vi "Configure Session.vi"(8 "error in":errorcluster, 11 "Plugin in":refnum<class "Sequencer with Output Values.lvclass">) -> (0 "error out":errorcluster, 3 "Plugin out":refnum<class "Sequencer with Output Values.lvclass">)   [LabVIEW 2024, in "Sequencer with Output Values.lvlib" / "Sequencer with Output Values.lvclass"]
uses:
  Sequencer with Output Values.lvclass
  C:/Program Files/National Instruments/LabVIEW 2024/vi.lib/FlexLogger/SDK/PluginSDK.lvlibp/PEFClasses/SDK/Processing Element/Processing Element.lvclass
  C:/Program Files/National Instruments/LabVIEW 2024/vi.lib/FlexLogger/SDK/PluginSDK.lvlibp/PEFClasses/SDK/Plugin/Plugin.lvclass
  Sequencer with Output Values.lvclass/Sequencer with Output Values.ctl
  <vilib>/FlexLogger/SDK/PluginSDK.lvlibp/PEFClasses/SDK/Producer Channel/Producer Channel.lvclass
  C:/Program Files/National Instruments/LabVIEW 2024/vi.lib/FlexLogger/SDK/PluginSDK.lvlibp/PEFClasses/SDK/Channel/Channel.lvclass
  <vilib>/FlexLogger/SDK/PluginSDK.lvlibp/PEFClasses/SDK/Processing Element/Read Alias.vi
  Global Strings.vi
  <vilib>/FlexLogger/SDK/PluginSDK.lvlibp/PEFClasses/SDK/Plugin/ParameterAccess/Read String.vi
  <vilib>/FlexLogger/SDK/PluginSDK.lvlibp/PEFClasses/SDK/Plugin/Plugin.lvclass
  C:/dev/niflexlogger-plugins/plugins/Sequencer with Output Values/source/Sequencer with Output Values/Sequencer with Output Values.lvclass
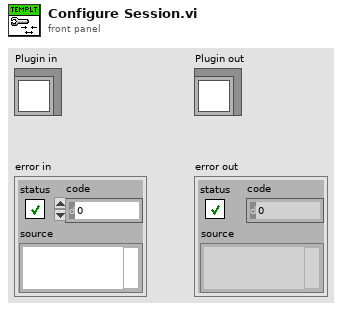
[diagram p1: front panel]
types:
  T1 = typedef "Sequencer with Output Values.lvlib/Sequencer with Output Values.lvclass/Params.ctl" = cluster{"Step Values":T2[], "Only Execute When Test Running":bool, "Reset Sequence When Test Starts":bool, "Current Sequence ID":u32, "Total Iterations":u32, "Current Step Start Timestamp":dbl, "Number of Sequence Steps":i32, "Num of Analog Channels":i32, "Num of Digital Channels":i32, "Delay Before Starting Sequence":dbl, "Show UI":bool, "Time Remaining":dbl, "Test Running":bool, "Pause Timestamp":dbl, "Default Analog Values":dbl[], "Default Digital Values":bool[]}
  T2 = typedef "Sequencer with Output Values.lvlib/Sequencer with Output Values.lvclass/Step Settings.ctl" = cluster{"Duration":dbl, "Mode":string, "Delay Between Values":dbl, "Analog Values":string[], "Digital Values":string[]}
  T3 = typedef "Sequencer with Output Values.lvlib/Sequencer with Output Values.lvclass/Cust UI.ctl" = refnum<vi>
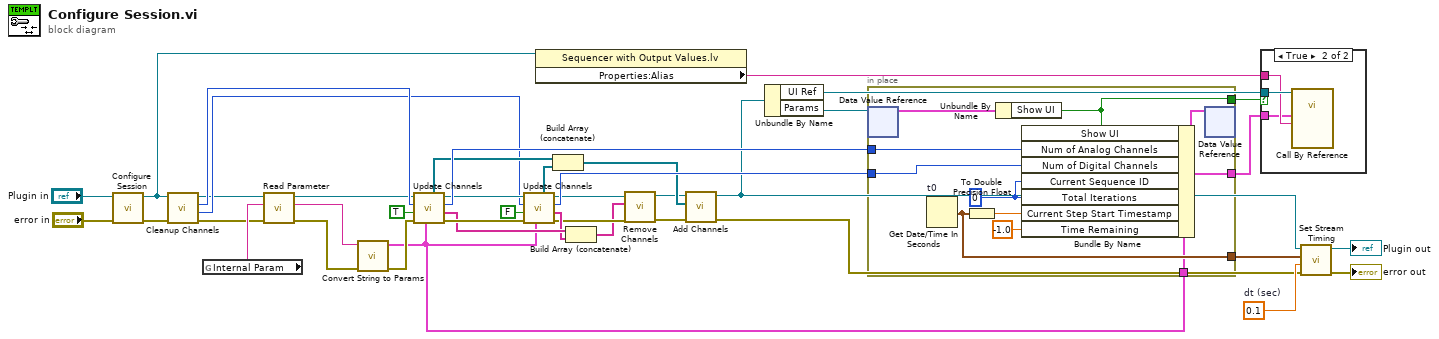
[diagram p0: block diagram]
diagram:
  w38 = 0.1  # dt (sec)
  n1 = call-parent "Configure Session.vi"("error in (no error)"="error in", "Processing Element in"="Plugin in") -> ("error out"=w17:errorcluster, "Processing Element out"=w8:refnum<class "Sequencer with Output Values.lvclass">)  [unwired: 8 in]
  n2 = call "Cleanup Channels.vi"("error in (no error)"=w17, "Plugin In"=w8) -> ("error out"=w13:errorcluster, "Num of Digital Channels"=w15:i32, "Num of Analog Channels"=w16:i32, "Plugin out"=w14:refnum<class "Sequencer with Output Values.lvclass">)  [unwired: 6 in]
  n3 = global read "Global Strings.vi" "Internal Param"() -> (w30:string)
  n4 = call-poly <vilib>:"Read Parameter.vi"("error in (no error)"=w13, "Name"=w30, "Plugin in"=w14) -> ("error out"=w18:errorcluster, "Value"=w3:string, "Plugin out"=w12:refnum<class "Sequencer with Output Values.lvclass">)  [unwired: 5 in, 1 out]
  n5 = call "Convert String to Params.vi"("error in (no error)"=w18, "String In"=w3) -> ("error out"=w29:errorcluster, "Param Out"=w4:T1)  [unwired: 8 in]
  n6 = call "Update Channels.vi"("Settings"=w4, "error in"=w29, "Analog"=TRUE, "Previous Number of Channels"=w16, "Plugin in"=w12) -> ("error out"=w32:errorcluster, "Channels to Remove"=w24:string[], "Updated Number of Channels"=w36:i32, "Plugin out"=w33:refnum<class "Sequencer with Output Values.lvclass">, "Channels to Add"=w27:refnum<class "Producer Channel.lvclass">[])  [unwired: 2 in]
  n7 = call "Update Channels.vi"("Settings"=w4, "error in"=w32, "Analog"=FALSE, "Previous Number of Channels"=w15, "Plugin in"=w33) -> ("error out"=w21:errorcluster, "Channels to Remove"=w23:string[], "Updated Number of Channels"=w35:i32, "Plugin out"=w22:refnum<class "Sequencer with Output Values.lvclass">, "Channels to Add"=w26:refnum<class "Producer Channel.lvclass">[])  [unwired: 2 in]
  n8 = property class="Sequencer with Output Values.lv"(reference=w8) -> ("Properties:Alias"=w10:string)  [unwired: 1 in, 2 out]
  n9 = Build Array (concatenate)(w27, w26) -> (w25:refnum<class "Producer Channel.lvclass">[])
  n10 = Build Array (concatenate)(w24, w23) -> (w1:string[])
  n11 = call-dynamic "Remove Channels.vi"("error in (no error)"=w21, "Unique Channel Identifiers to Delete"=w1, "Plugin in"=w22) -> ("error out"=w19:errorcluster, "Plugin out"=w20:refnum<class "Sequencer with Output Values.lvclass">)  [unwired: 7 in]
  n12 = call <vilib>:"Add Channels.vi"("error in (no error)"=w19, "Channels"=w25, "Plugin in"=w20) -> ("error out"=w2:errorcluster, "Plugin out"=w7:refnum<class "Sequencer with Output Values.lvclass">)  [unwired: 7 in]
  n13 = Unbundle By Name(w7) -> ("UI Ref"=w11:T3, "Params"=w9:refnum<data-value>)
  n14 = in-place {
    in-place-border: [w50] -> w37
    in-place-border: w36 -> [w48]
    in-place-border: w35 -> [w49]
    in-place-border: w4 -> [w47]
    in-place-border: [w45] -> w6
    in-place-border: [w44] -> w5
    w51 = u32 0 ("Current Sequence ID")
    n15 = in-place-dvr #1(w9) -> (w46:T1)  [unwired: 1 out]
    n16 = Get Date/Time In Seconds "t0"() -> (seconds since 1Jan1904=w50:timestamp)
    n17 = To Double Precision Float(number=w50) -> (double precision float=w42:dbl)
    n18 = Unbundle By Name(w46) -> ("Show UI"=w44:bool)
    n19 = Bundle By Name(cluster=w47, "Show UI"=w44, "Num of Analog Channels"=w48, "Num of Digital Channels"=w49, "Current Sequence ID"=w51, "Total Iterations"=w51, "Current Step Start Timestamp"=w42, "Time Remaining"=-1.0) -> (w45:T1)
    n20 = in-place-dvr #1(w45) -> ()  [unwired: 2 out]
  }
  n21 = case shown="True" w5 {
    tunnel: w11 -> [_ w54]
    tunnel: w10 -> [_ w53]
    tunnel: w6 -> [_ w52]
    frame False {
    }
    frame True {
      n22 = call-by-ref "?"(reference=w54, "Alias"=w53, "Init Settings In"=w52) -> ()  [unwired: 9 in, 4 out]
    }
  }
  n23 = call-dynamic "Set Stream Timing.vi"("error in (no error)"=w2, "dt(sec)"=w38, "Start Time"=w37, "Plugin in"=w7) -> ("error out"=→"error out":errorcluster, "Plugin out"=→"Plugin out":refnum<class "Sequencer with Output Values.lvclass">)  [unwired: 6 in]
